vi "Queue Comms Dequeue.vi"(8 "error in":errorcluster) -> (0 "error out":errorcluster, 3 "Data Out":T1={"Data"=variant, "Action"=enum."Error"})   [LabVIEW 2010, in "Sensor Console.lvlib"]
doc: "This VI dequeues data. Should be swapped\nif different comms method used."
uses:
  Sensor Console.lvlib
  Private Controls/Queue FG Action.ctl
  Private Controls/Sensor Action.ctl
  Private Controls/Sensor Data Cluster.ctl
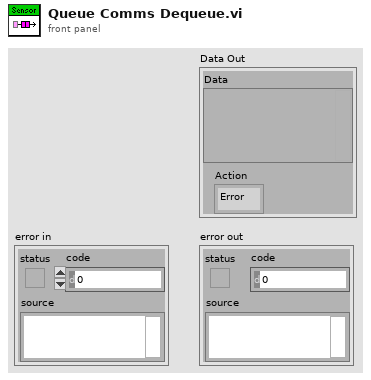
[diagram p1: front panel]
types:
  T1 = typedef "Sensor Console.lvlib/Sensor Data Cluster.ctl" = cluster{"Data":variant, "Action":T2}
  T2 = typedef "Sensor Console.lvlib/Sensor Action.ctl" = enum16{"Init", "Deposit", "Disburse", "Error", "Exit"}
  T3 = typedef "Sensor Console.lvlib/Queue FG Action.ctl" = enum16{"Release", "Get", "Set"}
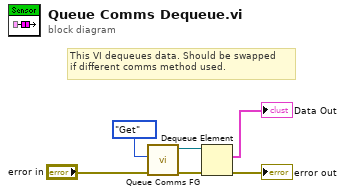
[diagram p0: block diagram]
diagram:
  # "This VI dequeues data. Should be swapped\nif different comms method used."
  n1 = call "Queue Comms FG.vi"("error in"="error in", "Action"=Queue_FG_Action."Get") -> ("error out"=w4:errorcluster, "Queue out"=w5:refnum<queue>)  [unwired: 8 in]
  n2 = Dequeue Element(queue=w5, error in (no error)=w4) -> (element=→"Data Out":T1, error out=→"error out":errorcluster)  [unwired: 1 in, 2 out]
